vi "Property Operator.vi"(7 "Command":T12, 8 "error in":errorcluster, 10 "User Input":T1, 11 "Data":T2) -> (0 "error out":errorcluster, 2 "User Input 2":T1, 3 "Data 2":T2)   [LabVIEW 2017]
uses:
  Ctrl/Property.ctl
  Ctrl/PhysicalChannel.ctl
  Ctrl/Bitfield.ctl
  Ctrl/Register.ctl
  Ctrl/ScaleType.ctl
  Ctrl/Scale.ctl
  Ctrl/EnumValue.ctl
  Ctrl/Enum.ctl
  Ctrl/Caps.ctl
  Ctrl/Data.ctl
  Ctrl/compond commands.ctl
  Ctrl/UserInput.ctl
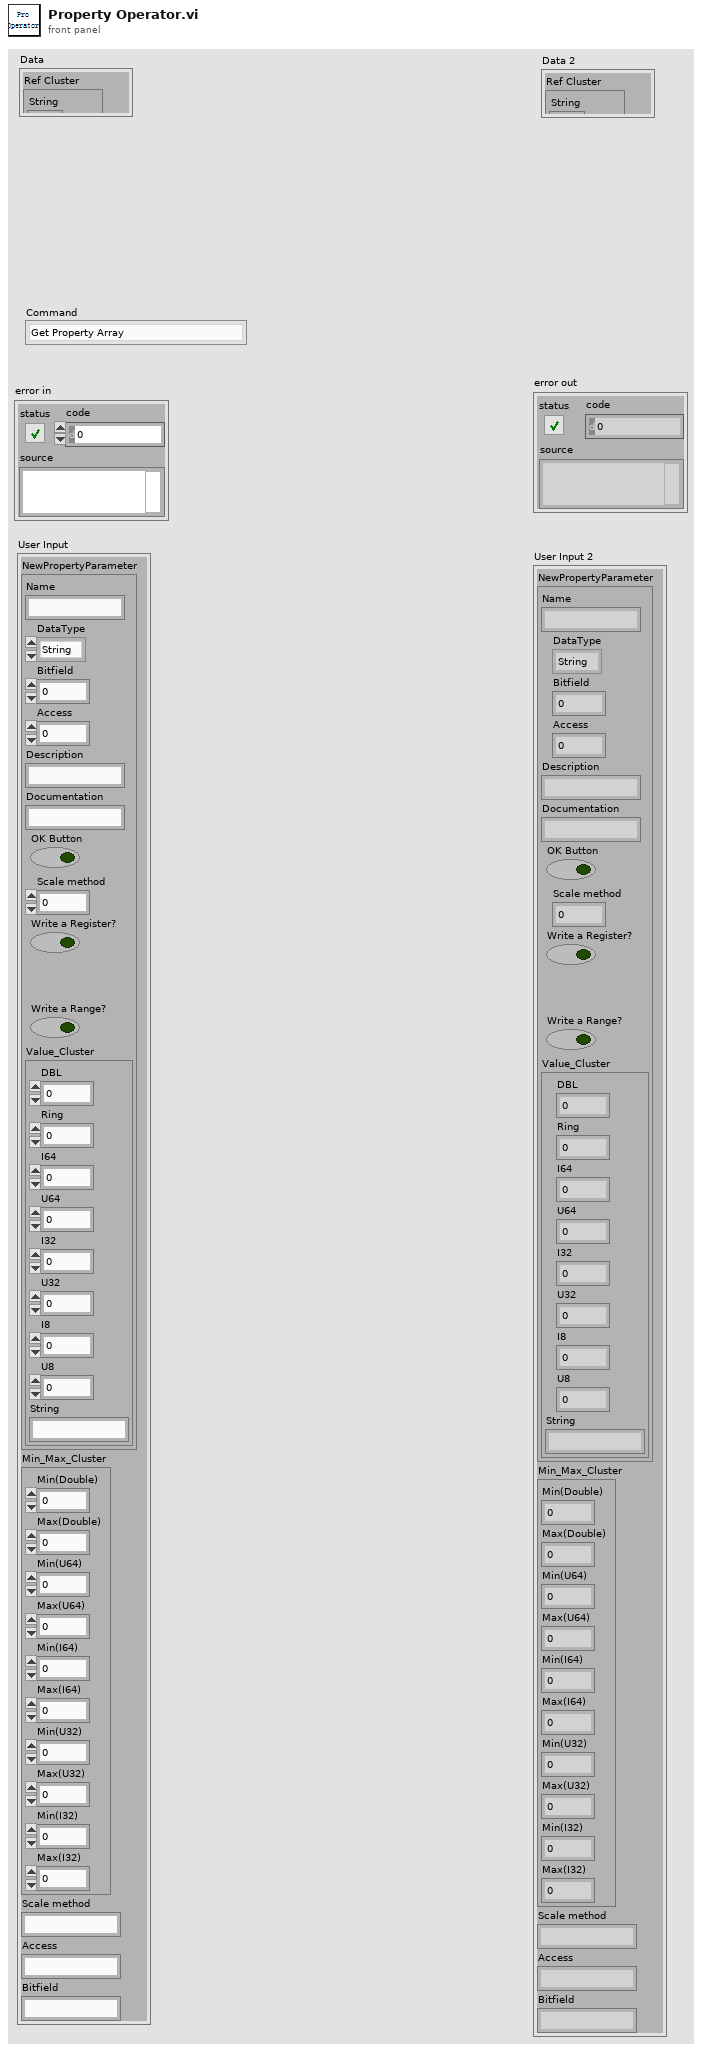
[diagram p1: front panel]
types:
  T1 = typedef "UserInput.ctl" = cluster{"NewPropertyParameter":cluster{"Name":string, "DataType":enum16{"String", "Double", "U64", "I64", "U32", "I32", "Bool"}, "Bitfield":u16, "Access":u16, "Description":string, "Documentation":string, "OK Button":bool, "Scale method":u16, "Write a Register?":bool, "Write a Range?":bool, "Value_Cluster":cluster{"DBL":dbl, "Ring":u16, "I64":i64, "U64":u64, "I32":i32, "U32":u32, "I8":i8, "U8":u8, "String":string}}, "Min_Max_Cluster":cluster{"Min(Double)":dbl, "Max(Double)":dbl, "Min(U64)":u64, "Max(U64)":u64, "Min(I64)":i64, "Max(I64)":i64, "Min(U32)":u32, "Max(U32)":u32, "Min(I32)":i32, "Max(I32)":i32}, "Scale method":string, "Access":string, "Bitfield":string}
  T2 = typedef "Data.ctl" = cluster{"Ref Cluster":cluster{"String":refnum<vi>, "U8":refnum<vi>, "I8":refnum<vi>, "U32":refnum<vi>, "I32":refnum<vi>, "U64":refnum<vi>, "I64":refnum<vi>, "Ring":refnum<vi>, "DBL":refnum<vi>, "Add":refnum<vi>, "Remove":refnum<vi>, "Property tree":refnum<vi>, "confirm":refnum<vi>}, "JSON Text":string, "Original JSON Text":string, "Caps":T3, "SLSC Output Tree":cluster{"Left Cell String":string, "Child Text":string[], "Child Tag":string, "Item Indent":i32, "Child Only?":bool, "Glyph Index":i32, "offline value":variant}[], "Ref Index and Control Type":cluster{"index":i32, "Datatype":string}, "Selected Type and name":cluster{"Selected Type":enum16{"Property", "Physical Channel", "Other"}, "Selected Property Name":string}, "Update whole Tree?":bool}
  T3 = typedef "Caps.ctl" = cluster{"properties":T4[], "physical channels":T5[], "registers":T6[], "scales":T8[], "enums":T10[], "productName":string}
  T4 = typedef "Property.ctl" = cluster{"name":string, "bitfield":string, "value":variant, "dataType":string, "min":variant, "max":variant, "scale":string, "access":string}
  T5 = typedef "PhysicalChannel.ctl" = cluster{"name":string, "properties":T4[]}
  T6 = typedef "Register.ctl" = cluster{"name":string, "address":i32, "size":i32, "bitfields":T7[], "initialValue":variant, "connectedProperties":string[]}
  T7 = typedef "Bitfield.ctl" = cluster{"name":string, "offset":i32, "size":i32, "signed":bool}
  T8 = typedef "Scale.ctl" = cluster{"name":string, "type":T9, "params":variant}
  T9 = typedef "ScaleType.ctl" = enum16{"NoScale", "Table", "Polynomial", "Linear"}
  T10 = typedef "Enum.ctl" = cluster{"name":string, "values":T11[]}
  T11 = typedef "EnumValue.ctl" = cluster{"name":string, "value":i32}
  T12 = typedef "compond commands.ctl" = enum16{"Get Property Array", "Get Physical Channel Property Array", "Get the Selected Position", "Get Property and Physical Channel Name", "Get Type and Value", "Make and Set a new Property", "Modify the Value", "Delete a Property"}
  T13 = cluster{"Physical Channel Index":i32, "Property Index":i32}
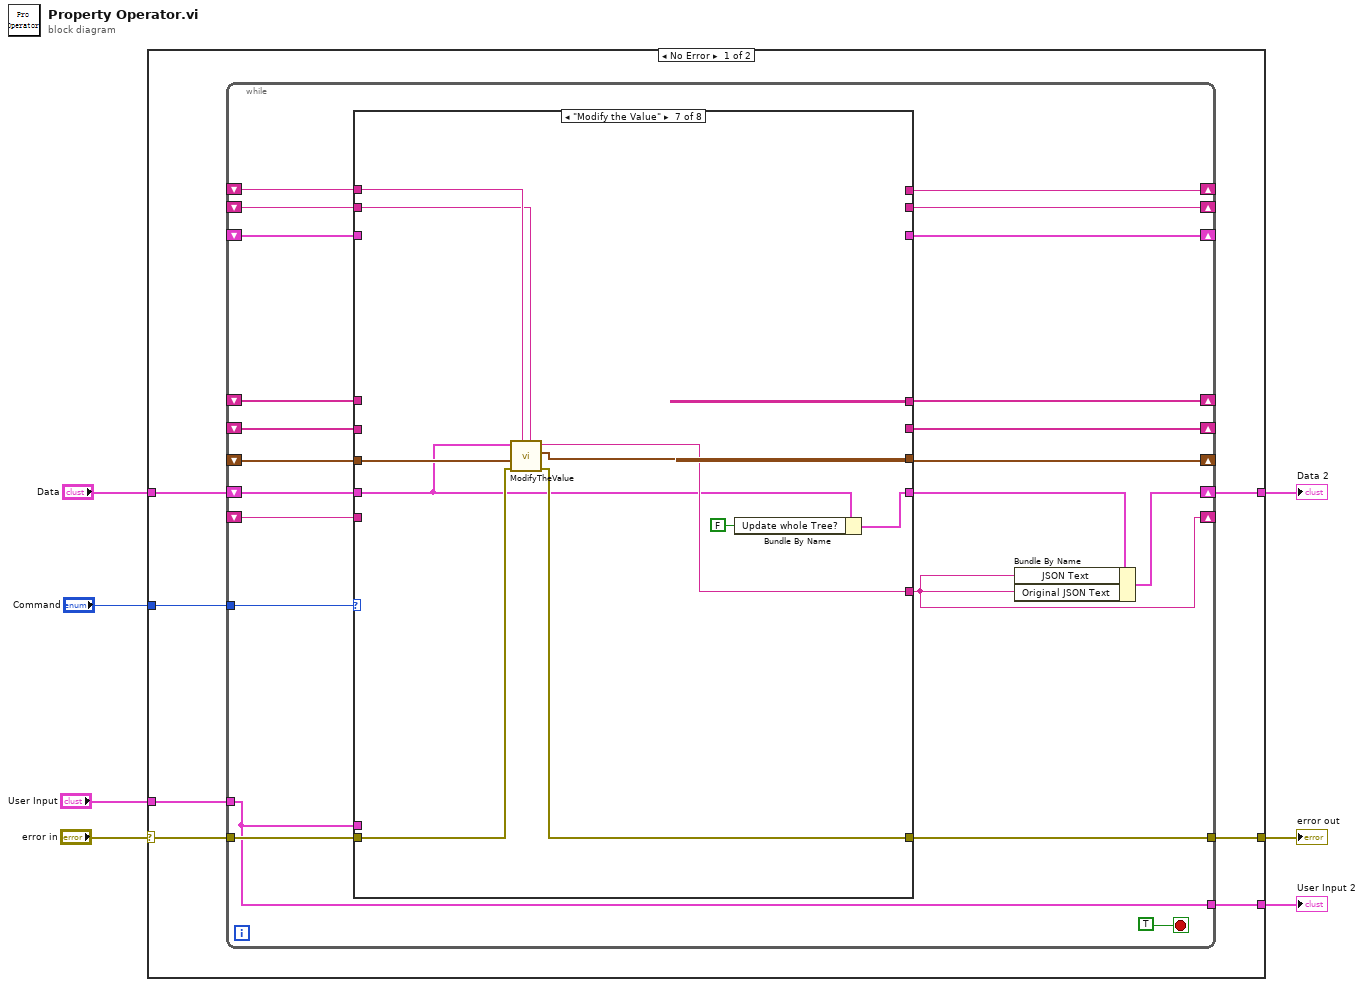
[diagram p0: block diagram]
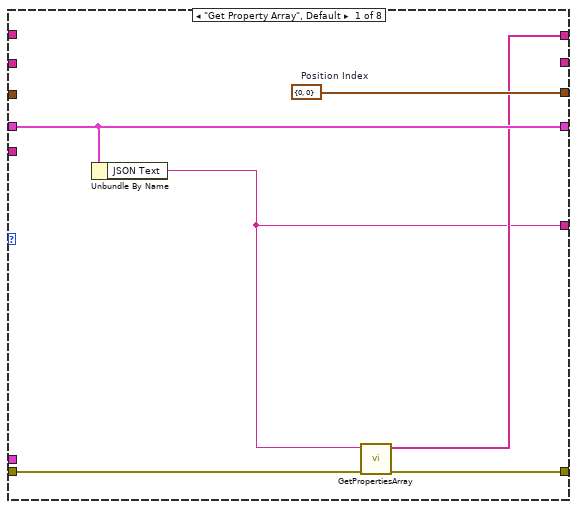
[diagram p2: hidden frame]
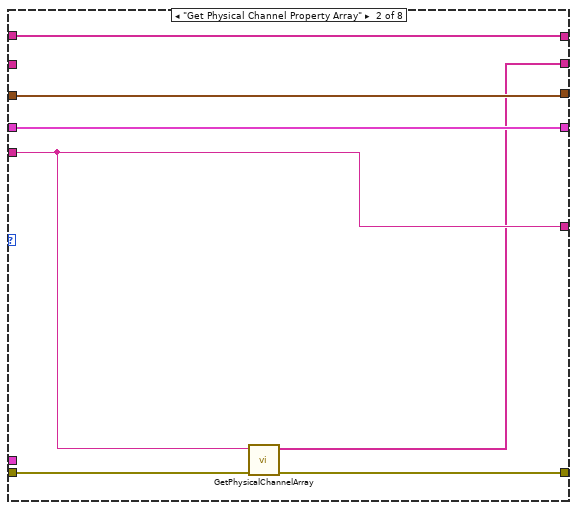
[diagram p3: hidden frame]
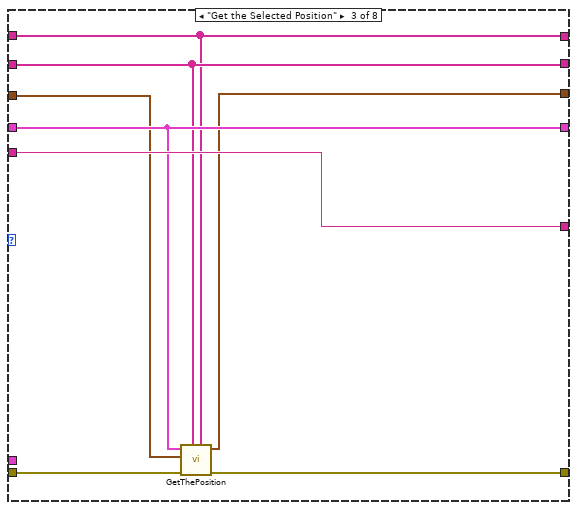
[diagram p4: hidden frame]
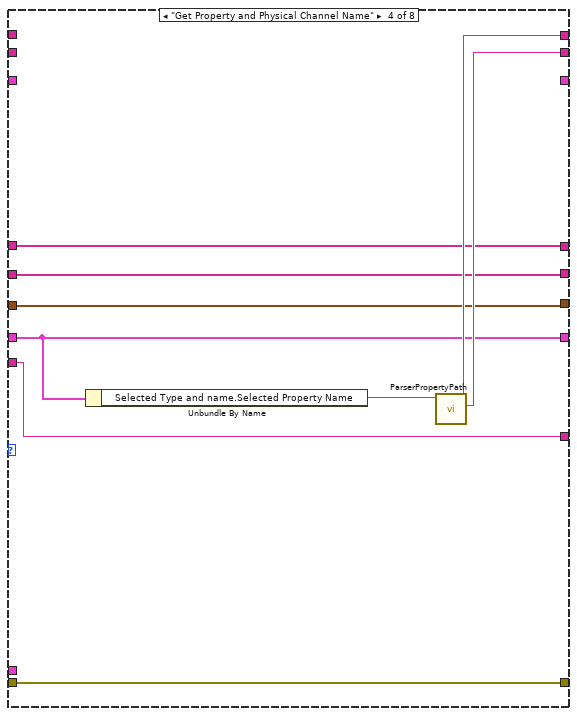
[diagram p5: hidden frame]
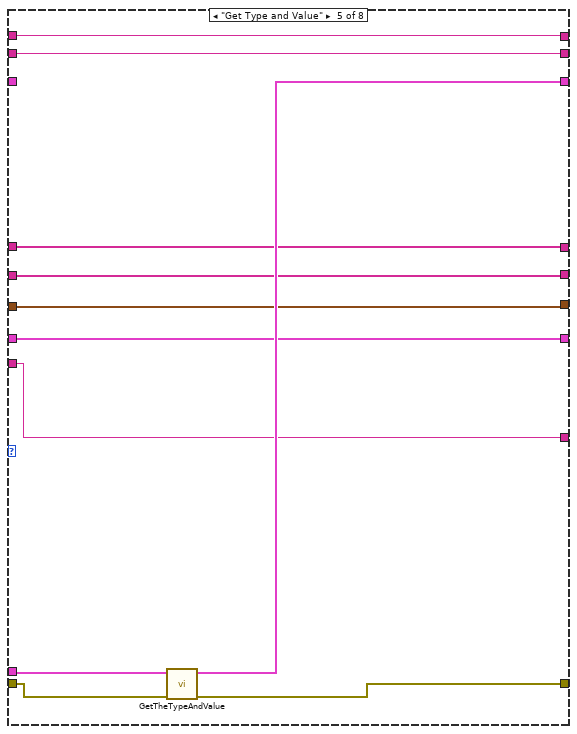
[diagram p6: hidden frame]
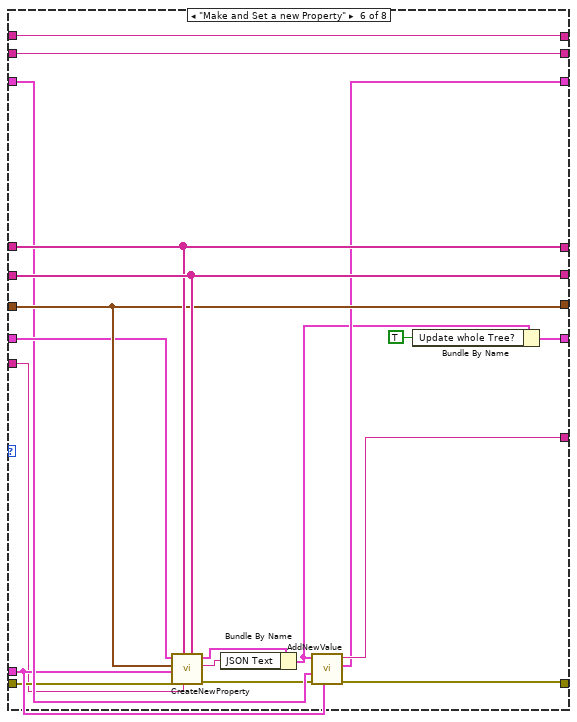
[diagram p7: hidden frame]
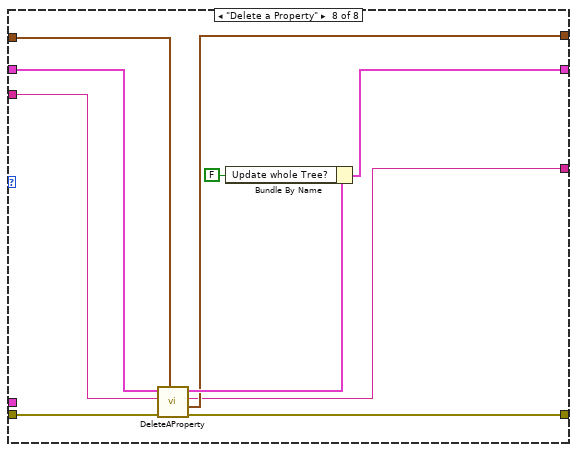
[diagram p8: hidden frame]
diagram:
  n1 = case shown="No Error" "error in" {
    selector: "error in" -> [w13 w119]
    tunnel: "Command" -> [w14 _]
    tunnel: [w12 w119] -> w5
    tunnel: "User Input" -> [w9 w117]
    tunnel: "Data" -> [w11 w118]
    tunnel: [w10 w118] -> w3
    tunnel: [w8 w117] -> w1
    frame No Error {
      n2 = while {
        tunnel: w14 -> [w35]
        tunnel: w13 -> [w32]
        shift-right: [w21] -> _
        shift-left: _ -> [w33]
        tunnel: [w30] -> w12
        shift-right: [w31] -> _
        shift-left: _ -> [w29]
        shift-right: [w28] -> _
        shift-left: _ -> [w27]
        shift-right: [w25] -> _
        shift-left: _ -> [w34]
        tunnel: w9 -> [w22]
        tunnel: [w22] -> w8
        shift-right: [w23] -> w10
        shift-left: w11 -> [w26]
        shift-right: [w20] -> _
        shift-left: _ -> [w18]
        shift-right: [w19] -> _
        shift-left: _ -> [w17]
        shift-right: [w16] -> _
        shift-left: _ -> [w15]
        stop <- TRUE stop-if-true
        n3 = case shown="\"Modify the Value\"" w35 {
          tunnel: w34 -> [_ w47 w53 w62 w69 w94 w106 w112]
          tunnel: w33 -> [_ w44 w57 w61 w67 w79 _ w113]
          tunnel: w32 -> [w40 w45 w50 w60 w76 w80 w105 w111]
          tunnel: [w38 w49 w54 w64 w71 w95 _ _] -> w31
          tunnel: [w39 w46 w51 w60 w75 w89 w102 w109] -> w30
          tunnel: [w37 w44 w57 w61 w67 w87 w104 w107] -> w21
          tunnel: w29 -> [_ w49 w54 w64 w71 w95 _ _]
          tunnel: [_ w43 w55 w63 w70 w96 _ _] -> w28
          tunnel: w27 -> [_ _ w55 w63 w70 w96 _ _]
          tunnel: w26 -> [w41 w48 w56 w59 w68 w93 w101 w114]
          tunnel: [w42 w47 w52 w62 w69 w94 w103 w108] -> w25
          tunnel: [w41 w48 w56 w59 w68 w81 w99 w115] -> w24
          tunnel: w22 -> [_ _ _ _ w77 w88 _ _]
          tunnel: [_ _ _ w66 w73 w85 _ _] -> w20
          tunnel: [_ _ _ w65 w72 w84 _ _] -> w19
          tunnel: w18 -> [_ _ _ _ w73 w85 w98 _]
          tunnel: w17 -> [_ _ _ _ w72 w84 w97 _]
          tunnel: [_ _ _ _ w74 w86 _ _] -> w16
          tunnel: w15 -> [_ _ _ _ _ w92 _ _]
          frame "Get Property Array", Default {
            w42 = T13 {"Physical Channel Index"=0, "Property Index"=0}  # Position Index
            n4 = Unbundle By Name(w41) -> ("JSON Text"=w37:string)
            n5 = call "GetPropertiesArray.vi"("error in (no error)"=w40, "JSON Text"=w37) -> ("error out"=w39:errorcluster, "Properties Array"=w38:string[])  [unwired: 8 in]
          }
          frame "Get Physical Channel Property Array" {
            n6 = call "GetPhysicalChannelArray.vi"("error in (no error)"=w45, "JSON Text"=w44) -> ("error out"=w46:errorcluster, "PhysicalChannels Array"=w43:string[])  [unwired: 8 in]
          }
          frame "Get the Selected Position" {
            n7 = call "GetThePosition.vi"("Property Array"=w54, "Physical Channel Array"=w55, "error IO"=w50, "Position Index In"=w53, "Data in"=w56) -> ("error out"=w51:errorcluster, "Position Index Out"=w52:T13)  [unwired: 5 in]
          }
          frame "Get Property and Physical Channel Name" {
            n8 = Unbundle By Name(w59) -> ("Selected Type and name.Selected Property Name"=w58:string)
            n9 = call "ParserPropertyPath.vi"("property"=w58) -> ("name"=w65:string, "pyhsical channel"=w66:string)  [unwired: 7 in]
          }
          frame "Get Type and Value" {
            n10 = call "GetTheTypeAndValue.vi"("error in (no error)"=w76, "Data Cluster"=w77) -> ("error out"=w75:errorcluster, "DataType and Value"=w74:cluster{"Type":string, "Value":variant})  [unwired: 8 in]
          }
          frame "Make and Set a new Property" {
            n11 = call "CreateNewProperty.vi"("Physical Channels Array"=w96, "JSON Text In"=w79, "Properties Array"=w95, "error IO"=w80, "User Input"=w88, "Position Index"=w94, "Data"=w93) -> ("error out"=w90:errorcluster, "JSON Text Out"=w78:string, "Data Out"=w91:T2)  [unwired: 2 in]
            n12 = Bundle By Name(cluster=w91, "JSON Text"=w78) -> (w83:T2)
            n13 = call "AddNewValue.vi"("Data Cluster"=w88, "error IO"=w90, "DataType and Value"=w92, "Data"=w83) -> ("error IO Out"=w89:errorcluster, "DataType and Value Out"=w86:cluster{"Type":string, "Value":variant}, "JSON Text Out"=w87:string)  [unwired: 5 in]
            n14 = Bundle By Name(cluster=w83, "Update whole Tree?"=TRUE) -> (w81:T2)
          }
          frame "Modify the Value" {
            n15 = call "ModifyTheValue.vi"("property name"=w97, "physical channel name"=w98, "error in (no error)"=w105, "Physical Channel Index Cluster"=w106, "Data"=w101) -> ("error out"=w102:errorcluster, "Physical Channel Index Cluster Out"=w103:T13, "JSON Text Out"=w104:string)  [unwired: 4 in]
            n16 = Bundle By Name(cluster=w101, "Update whole Tree?"=FALSE) -> (w99:T2)
          }
          frame "Delete a Property" {
            n17 = call "DeleteAProperty.vi"("Position Index"=w112, "error IO"=w111, "JSON Text"=w113, "Data"=w114) -> ("error out"=w109:errorcluster, "Position Index Out"=w108:T13, "JSON Text out"=w107:string, "Data Out"=w110:T2)  [unwired: 4 in]
            n18 = Bundle By Name(cluster=w110, "Update whole Tree?"=FALSE) -> (w115:T2)
          }
        }
        n19 = Bundle By Name(cluster=w24, "JSON Text"=w21, "Original JSON Text"=w21) -> (w23:T2)
      }
    }
    frame Error {
    }
  }
  "error out" <- w5
  "Data 2" <- w3
  "User Input 2" <- w1
